vi "MCL Get Tip Tilt Theta Y.vi"(11 "handle":i32) -> (3 "function return":dbl)   [LabVIEW 2017, in "Madlib.lvlib"]
doc: "MADLIB_API double MCL_GetTipTiltThetaY(int handle);"
uses:
  Madlib.lvlib
  Madlib.dll
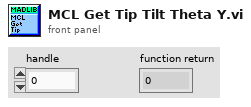
[diagram p1: front panel]
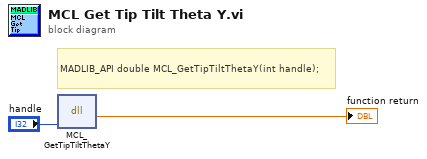
[diagram p0: block diagram]
diagram:
  # "MADLIB_API\tdouble\tMCL_GetTipTiltThetaY(int handle);"
  n1 = dll-call lib="C:/Users/francesco/dev/pump-probe/Piezo/lvlib/Madlib.*" fn="MCL_GetTipTiltThetaY"("handle"="handle") -> (→"function return":dbl)  [unwired: 4 in, 2 out]
